vi "ThermoV_ControlSweep_2VO_VG2_nomean_DC_170909.vi"() -> ()   [LabVIEW 2013]
panel:
  out "VG indicate":dbl[](array[numeric]) format="%#.6f"
  out "time/(60*13) indicator":dbl
  out "VGate Mod10 indicator":dbl
  in  "Operate HVpp\nOutput Timer":bool caption="Reset"
  out "modular 13":dbl
  in  "Number of seconds for \neach HVpp case state":dbl=30.0
  out "Elapsed Time (s)":dbl
  out "DC Value":dbl[](array[numeric]) format="%#.6f"
  in  "Saving Avg?":bool
  in  "Filename":path=path "trial_1.lvm"
  in  "STOP":bool
  in  "Save Waveform":bool
  out "Peak2Peak V":dbl[](array[numeric])
  out "Waveform Chart":dynamicdata(graph)
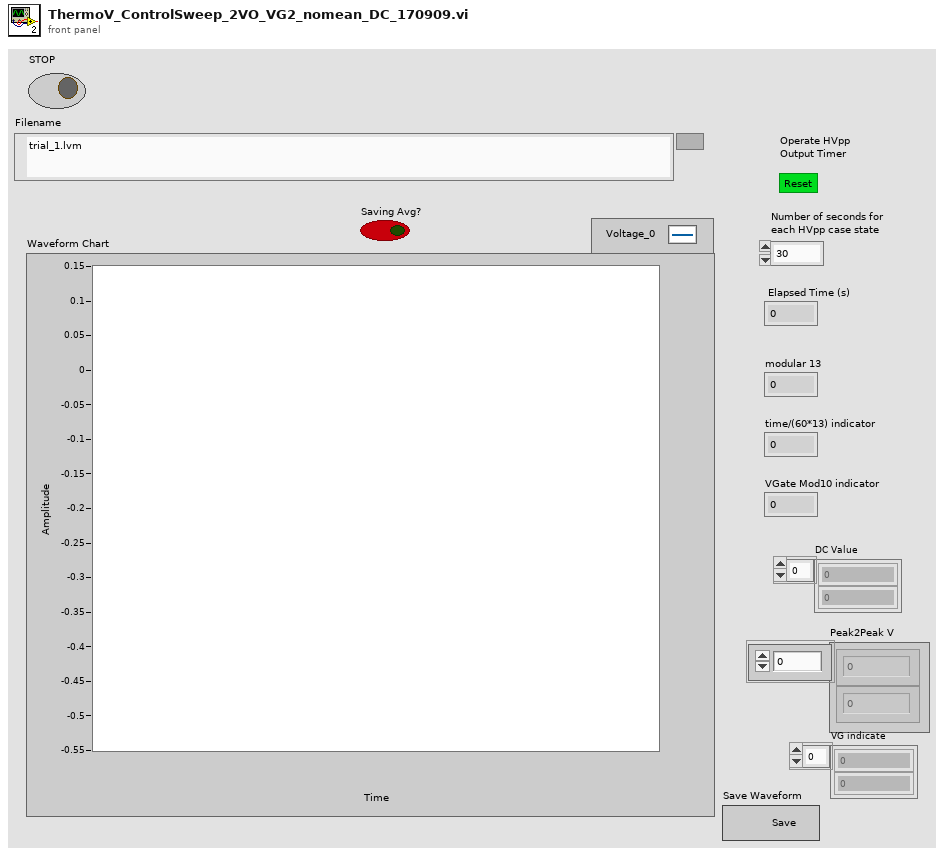
[diagram p1: front panel]
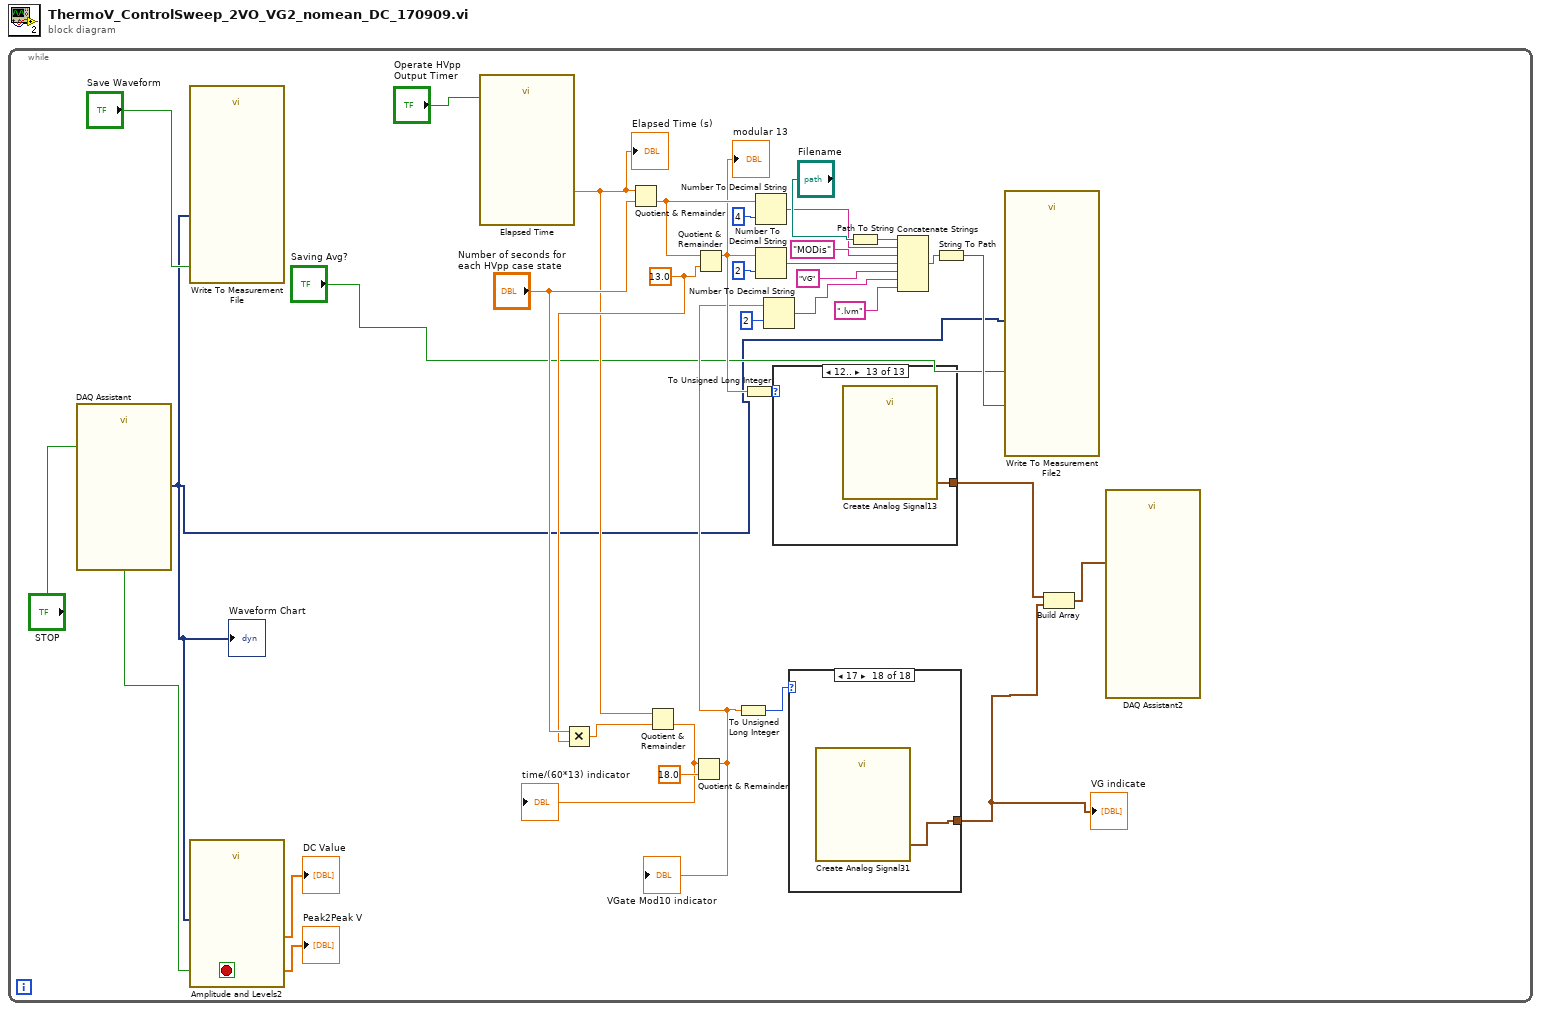
[diagram p0: block diagram]
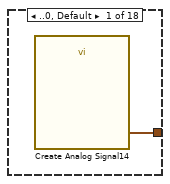
[diagram p2: hidden frame]
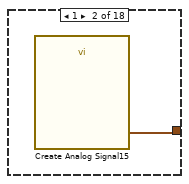
[diagram p3: hidden frame]
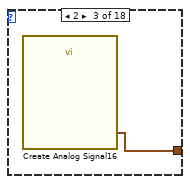
[diagram p4: hidden frame]
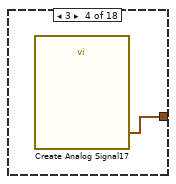
[diagram p5: hidden frame]
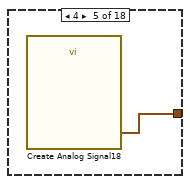
[diagram p6: hidden frame]
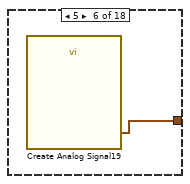
[diagram p7: hidden frame]
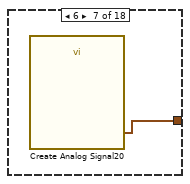
[diagram p8: hidden frame]
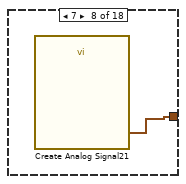
[diagram p9: hidden frame]
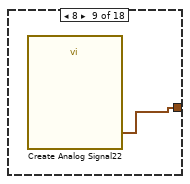
[diagram p10: hidden frame]
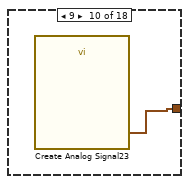
[diagram p11: hidden frame]
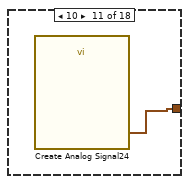
[diagram p12: hidden frame]
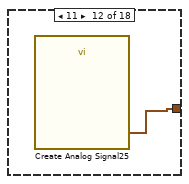
[diagram p13: hidden frame]
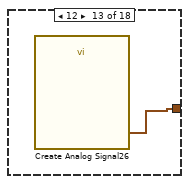
[diagram p14: hidden frame]
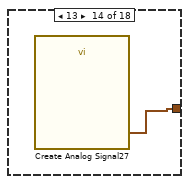
[diagram p15: hidden frame]
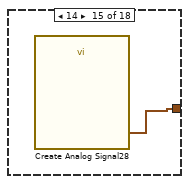
[diagram p16: hidden frame]
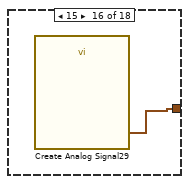
[diagram p17: hidden frame]
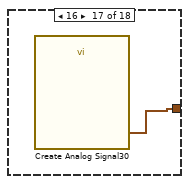
[diagram p18: hidden frame]
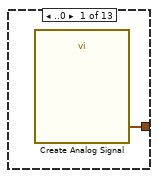
[diagram p19: hidden frame]
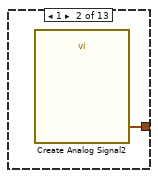
[diagram p20: hidden frame]
diagram:
  n1 = while {
    stop <- w35 stop-if-true
    w15 = 13.0 ("y")
    n2 = call "DAQ Assistant"("stop (F)"="STOP") -> ("data"=w2:dynamicdata, "stopped"=w35:bool)  [unwired: 15 in, 2 out]
    "Waveform Chart" <- w2
    n3 = call "Write To Measurement File"("Signals"=w2, "Enable"="Save Waveform") -> ()  [unwired: 15 in, 3 out]
    n4 = call "Amplitude and Levels2"("input signals"=w2) -> ("dc"=→"DC Value":dbl[], "peak-peak"=→"Peak2Peak V":dbl[])  [unwired: 15 in, 2 out]
    n5 = call "Elapsed Time"("Reset"="Operate HVpp\nOutput Timer") -> ("Elapsed Time (s)"=w14:dbl)  [unwired: 11 in, 7 out]
    "Elapsed Time (s)" <- w14
    n6 = Multiply(x="Number of seconds for \neach HVpp case state", y=w15) -> (x*y=w17:dbl)
    n7 = Quotient & Remainder(x=w14, y="Number of seconds for \neach HVpp case state") -> (floor(x/y)=w24:dbl)  [unwired: 1 out]
    n8 = Quotient & Remainder(x=w14, y=w17) -> (floor(x/y)=w8:dbl)  [unwired: 1 out]
    "time/(60*13) indicator" <- w8
    n9 = Quotient & Remainder(x=w8, y=18.0) -> (x-y*floor(x/y)=w7:dbl)  [unwired: 1 out]
    "VGate Mod10 indicator" <- w7
    n10 = Quotient & Remainder(x=w24, y=w15) -> (x-y*floor(x/y)=w20:dbl)  [unwired: 1 out]
    "modular 13" <- w20
    n11 = To Unsigned Long Integer(number=w7) -> (unsigned 32bit integer=w13:u32)
    n12 = To Unsigned Long Integer(number=w20) -> (unsigned 32bit integer=w30:u32)
    n13 = Number To Decimal String(number=w24, width (-)=i16 4) -> (decimal integer string=w23:string)
    n14 = Number To Decimal String(number=w20, width (-)=i16 2) -> (decimal integer string=w19:string)
    n15 = Number To Decimal String(number=w7, width (-)=i16 2) -> (decimal integer string=w10:string)
    n16 = case shown="12.." w30 {
      tunnel: [w54 w55 w56 w57 w58 w59 w60 w61 w62 w63 w64 w65 w66] -> w6
      frame ..0 {
        n17 = call "Create Analog Signal"() -> ("DC signal"=w54:waveform(dbl))  [unwired: 18 in, 1 out]
      }
      frame 1 {
        n18 = call "Create Analog Signal2"() -> ("DC signal"=w55:waveform(dbl))  [unwired: 18 in, 1 out]
      }
      frame 2 {
        n19 = call "Create Analog Signal3"() -> ("DC signal"=w56:waveform(dbl))  [unwired: 18 in, 1 out]
      }
      frame 3 {
        n20 = call "Create Analog Signal4"() -> ("DC signal"=w57:waveform(dbl))  [unwired: 18 in, 1 out]
      }
      frame 4 {
        n21 = call "Create Analog Signal5"() -> ("DC signal"=w58:waveform(dbl))  [unwired: 18 in, 1 out]
      }
      frame 5 {
        n22 = call "Create Analog Signal6"() -> ("DC signal"=w59:waveform(dbl))  [unwired: 18 in, 1 out]
      }
      frame 6 {
        n23 = call "Create Analog Signal7"() -> ("DC signal"=w60:waveform(dbl))  [unwired: 18 in, 1 out]
      }
      frame 7 {
        n24 = call "Create Analog Signal8"() -> ("DC signal"=w61:waveform(dbl))  [unwired: 18 in, 1 out]
      }
      frame 8 {
        n25 = call "Create Analog Signal9"() -> ("DC signal"=w62:waveform(dbl))  [unwired: 18 in, 1 out]
      }
      frame 9 {
        n26 = call "Create Analog Signal10"() -> ("DC signal"=w63:waveform(dbl))  [unwired: 18 in, 1 out]
      }
      frame 10 {
        n27 = call "Create Analog Signal11"() -> ("DC signal"=w64:waveform(dbl))  [unwired: 18 in, 1 out]
      }
      frame 11 {
        n28 = call "Create Analog Signal12"() -> ("DC signal"=w65:waveform(dbl))  [unwired: 18 in, 1 out]
      }
      frame 12.. {
        n29 = call "Create Analog Signal13"() -> ("DC signal"=w66:waveform(dbl))  [unwired: 18 in, 1 out]
      }
    }
    n30 = case shown="17" w13 {
      tunnel: [w36 w37 w38 w39 w40 w41 w42 w43 w44 w45 w46 w47 w48 w49 w50 w51 w52 w53] -> w1
      frame ..0, Default {
        n31 = call "Create Analog Signal14"() -> ("DC signal"=w36:waveform(dbl))  [unwired: 18 in, 1 out]
      }
      frame 1 {
        n32 = call "Create Analog Signal15"() -> ("DC signal"=w37:waveform(dbl))  [unwired: 18 in, 1 out]
      }
      frame 2 {
        n33 = call "Create Analog Signal16"() -> ("DC signal"=w38:waveform(dbl))  [unwired: 18 in, 1 out]
      }
      frame 3 {
        n34 = call "Create Analog Signal17"() -> ("DC signal"=w39:waveform(dbl))  [unwired: 18 in, 1 out]
      }
      frame 4 {
        n35 = call "Create Analog Signal18"() -> ("DC signal"=w40:waveform(dbl))  [unwired: 18 in, 1 out]
      }
      frame 5 {
        n36 = call "Create Analog Signal19"() -> ("DC signal"=w41:waveform(dbl))  [unwired: 18 in, 1 out]
      }
      frame 6 {
        n37 = call "Create Analog Signal20"() -> ("DC signal"=w42:waveform(dbl))  [unwired: 18 in, 1 out]
      }
      frame 7 {
        n38 = call "Create Analog Signal21"() -> ("DC signal"=w43:waveform(dbl))  [unwired: 18 in, 1 out]
      }
      frame 8 {
        n39 = call "Create Analog Signal22"() -> ("DC signal"=w44:waveform(dbl))  [unwired: 18 in, 1 out]
      }
      frame 9 {
        n40 = call "Create Analog Signal23"() -> ("DC signal"=w45:waveform(dbl))  [unwired: 18 in, 1 out]
      }
      frame 10 {
        n41 = call "Create Analog Signal24"() -> ("DC signal"=w46:waveform(dbl))  [unwired: 18 in, 1 out]
      }
      frame 11 {
        n42 = call "Create Analog Signal25"() -> ("DC signal"=w47:waveform(dbl))  [unwired: 18 in, 1 out]
      }
      frame 12 {
        n43 = call "Create Analog Signal26"() -> ("DC signal"=w48:waveform(dbl))  [unwired: 18 in, 1 out]
      }
      frame 13 {
        n44 = call "Create Analog Signal27"() -> ("DC signal"=w49:waveform(dbl))  [unwired: 18 in, 1 out]
      }
      frame 14 {
        n45 = call "Create Analog Signal28"() -> ("DC signal"=w50:waveform(dbl))  [unwired: 18 in, 1 out]
      }
      frame 15 {
        n46 = call "Create Analog Signal29"() -> ("DC signal"=w51:waveform(dbl))  [unwired: 18 in, 1 out]
      }
      frame 16 {
        n47 = call "Create Analog Signal30"() -> ("DC signal"=w52:waveform(dbl))  [unwired: 18 in, 1 out]
      }
      frame 17 {
        n48 = call "Create Analog Signal31"() -> ("DC signal"=w53:waveform(dbl))  [unwired: 18 in, 1 out]
      }
    }
    "VG indicate" <- w1
    n49 = Path To String(path="Filename") -> (string=w26:string)
    n50 = Concatenate Strings(w26, w23, "MODis" ("string"), w19, "VG" ("string"), w10, ".lvm" ("string")) -> (w27:string)
    n51 = String To Path(string=w27) -> (path=w28:path)
    n52 = call "Write To Measurement File2"("Signals"=w2, "Enable"="Saving Avg?", "Filename"=w28) -> ()  [unwired: 14 in, 3 out]
    n53 = Build Array(w6, w1) -> (w5:waveform(dbl)[])
    n54 = call "DAQ Assistant2"("data"=w5) -> ()  [unwired: 16 in, 3 out]
  }
